vi "Design IIR filter for N Waveforms.vi"(4 "Optional Filter Specifications":T4 {"PB Gain" format="%0.2f"; "SB Gain" format="%0.2f"; "Lower SB" format="%0.2p"; "Upper SB" format="%0.2f"; "Lower PB" format="%0.2p"; "Upper PB" format="%0.2f"}, 6 "Filter specifications":T5 {"PB Ripple" format="%0.2f"; "Lower Fc" format="%0.2p"; "SB Attenuation" format="%0.2f"; "Upper Fc" format="%0.2p"}, 7 "Reset history":bool, 8 "error in":errorcluster, 10 "filter structure option":T1=10 items=["IIR 2nd Order"=0, "IIR 4th Order"=1, "Auto Select"=10], 11 "arrdt":dbl[](array[numeric]) format="%0.2f") -> (0 "error out":errorcluster, 1 "IIR Filter Cluster":T2 {"Forward Coefficients" format="%0.2f"; "Reverse Coefficients" format="%0.2f"}, 3 "Filter Information":T3 {"phase H(w)"."df" format="%0.2f"; "phase H(w)"."f0" format="%0.2f"; "phase H(w)"."Phase H(w)" format="%0.2f"; "magnitude H(w)"."df" format="%0.2f"; "magnitude H(w)"."f0" format="%0.2f"; "magnitude H(w)"."Mag H(w)" format="%0.2f"}, 5 "reset filters":bool)   [LabVIEW 2020, in "NI_MAPro.lvlib"]
uses:
  NI_MAPro.lvlib
  Filter Structure Type.ctl
  NI_MABase.lvlib
  NI_AALBase.lvlib
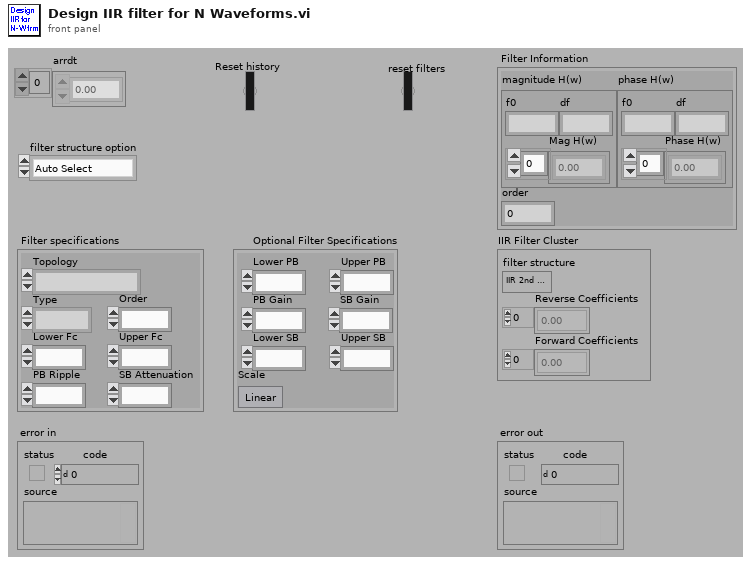
[diagram p1: front panel]
types:
  T1 = typedef "NI_AALBase.lvlib/Filter Structure Type.ctl" = u16
  T2 = cluster{"filter structure":enum32{"IIR 2nd Order", "IIR 4th Order"}, "Reverse Coefficients":dbl[], "Forward Coefficients":dbl[]}
  T3 = cluster{"magnitude H(w)":cluster{"f0":dbl, "df":dbl, "Mag H(w)":dbl[]}, "phase H(w)":cluster{"f0":dbl, "df":dbl, "Phase H(w)":dbl[]}, "order":i32}
  T4 = cluster{"Lower PB":dbl, "Upper PB":dbl, "Lower SB":dbl, "Upper SB":dbl, "PB Gain":dbl, "SB Gain":dbl, "Scale":bool}
  T5 = cluster{"Topology":enum16{"Off", "Butterworth", "Chebyshev", "Inverse Chebyshev", "Elliptic", "Bessel"}, "Type":enum16{"Lowpass", "Highpass", "Bandpass", "Bandstop"}, "Order":i32, "Lower Fc":dbl, "Upper Fc":dbl, "PB Ripple":dbl, "SB Attenuation":dbl}
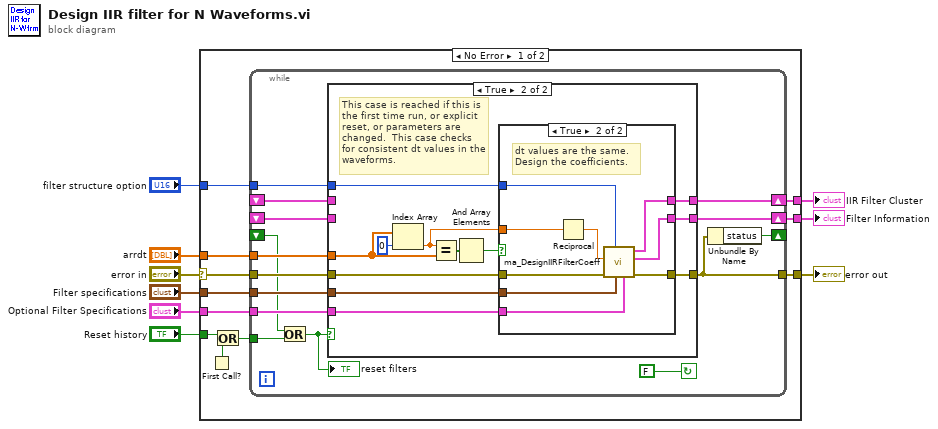
[diagram p0: block diagram]
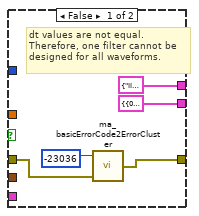
[diagram p3: hidden frame]
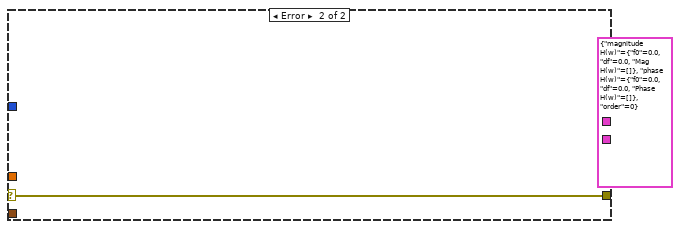
[diagram p4: hidden frame]
diagram:
  n1 = case shown="No Error" "error in" {
    selector: "error in" -> [w19 w67]
    tunnel: [w20 w67] -> w9
    tunnel: [w18 T3 {"magnitude H(w)"={"f0"=0.0, "df"=0.0, "Mag H(w)"=[]}, "phase H(w)"={"f0"=0.0, "df"=0.0, "Phase H(w)"=[]}, "order"=0} ("Filter Information")] -> w7
    tunnel: [w17 T2 {"filter structure"=enum."IIR 2nd Order", "Reverse Coefficients"=[], "Forward Coefficients"=[]} ("IIR Filter Cluster")] -> w6
    tunnel: "Optional Filter Specifications" -> [w16 _]
    tunnel: "Filter specifications" -> [w15 _]
    tunnel: "arrdt" -> [w14 _]
    tunnel: "filter structure option" -> [w13 _]
    tunnel: "Reset history" -> [w11 _]
    frame No Error {
      n2 = First Call?() -> (First Call?: T/F=w12:bool)
      n3 = Or(x=w11, y=w12) -> (x .or. y?=w10:bool)
      n4 = while {
        tunnel: w14 -> [w28]
        tunnel: w15 -> [w31]
        tunnel: w16 -> [w30]
        tunnel: w19 -> [w27]
        tunnel: [w25] -> w20
        shift-left: _ -> [w32]
        shift-right: [w33] -> w18
        shift-left: _ -> [w35]
        shift-right: [w29] -> w17
        tunnel: w10 -> [w23]
        shift-right: [w24] -> _
        shift-left: _ -> [w26]
        tunnel: w13 -> [w21]
        stop <- FALSE continue-if-true
        n5 = Or(x=w26, y=w23) -> (x .or. y?=w22:bool)
        "reset filters" <- w22
        n6 = case shown="True" w22 {
          tunnel: w35 -> [w38 _]
          tunnel: [w37 w50] -> w33
          tunnel: w32 -> [w37 _]
          tunnel: [w38 w49] -> w29
          tunnel: [w36 w48] -> w25
          tunnel: w28 -> [_ w41]
          tunnel: w31 -> [_ w47]
          tunnel: w30 -> [_ w46]
          tunnel: w27 -> [w36 w45]
          tunnel: w21 -> [_ w39]
          frame False {
            # "No change in parameters, no reset, and not the first time run."
          }
          frame True {
            # "This case is reached if this is the first time run, or explicit reset, or parameters are changed.  This case checks for consistent dt values in the waveforms."
            n7 = Index Array(array=w41, index=0 ("Index")) -> (element=w40:dbl)
            n8 = Equal?(x=w40, y=w41) -> (x = y?=w43:bool[])
            n9 = And Array Elements(Boolean array=w43) -> (logical AND=w42:bool)
            n10 = case shown="True" w42 {
              tunnel: [T3 {"magnitude H(w)"={"f0"=0.0, "df"=0.0, "Mag H(w)"=[]}, "phase H(w)"={"f0"=0.0, "df"=0.0, "Phase H(w)"=[]}, "order"=0} ("Filter Information") w57] -> w50
              tunnel: [T2 {"filter structure"=enum."IIR 2nd Order", "Reverse Coefficients"=[], "Forward Coefficients"=[]} ("IIR Filter Cluster") w64] -> w49
              tunnel: [w51 w63] -> w48
              tunnel: w47 -> [_ w62]
              tunnel: w46 -> [_ w59]
              tunnel: w45 -> [w52 w61]
              tunnel: w40 -> [_ w58]
              tunnel: w39 -> [_ w56]
              frame False {
                # "dt values are not equal.  \nTherefore, one filter cannot be \ndesigned for all waveforms."
                n11 = call "ma_basicErrorCode2ErrorCluster.vi"("error in (no error)"=w52, "Error Code"=-23036) -> ("error out"=w51:errorcluster)  [unwired: 1 in]
              }
              frame True {
                # "dt values are the same.  \nDesign the coefficients."
                n12 = Reciprocal(x=w58) -> (1/x=w60:dbl)
                n13 = call "ma_DesignIIRFilterCoeff.vi"("Optional Filter Specifications"=w59, "Filter specifications"=w62, "filter structure option"=w56, "error in (no error)"=w61, "Sampling Frequency"=w60) -> ("error out"=w63:errorcluster, "Filter Information"=w57:T3, "IIR Filter Cluster"=w64:T2)  [unwired: 4 in]
              }
            }
          }
        }
        n14 = Unbundle By Name(w25) -> ("status"=w24:bool)
      }
    }
    frame Error {
    }
  }
  "error out" <- w9
  "IIR Filter Cluster" <- w6
  "Filter Information" <- w7
